vi "Get_IP_Number.vi"() -> (0 "Computer Name":string, 1 "IP Number":string)   [LabVIEW 2013]
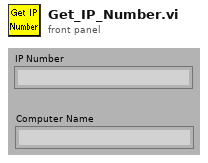
[diagram p1: front panel]
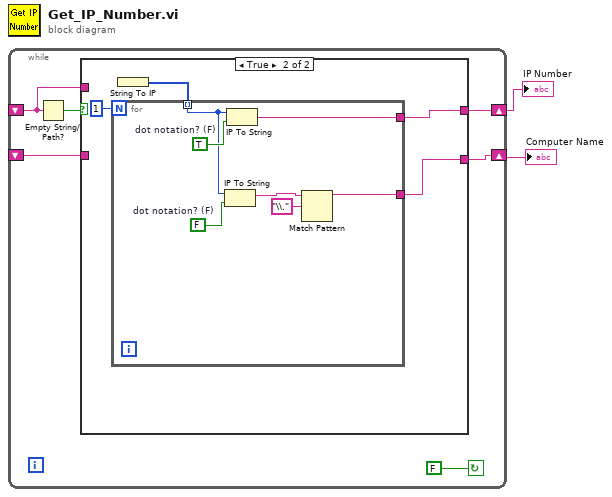
[diagram p0: block diagram]
diagram:
  n1 = while {
    shift-left: _ -> [w7]
    shift-right: [w8] -> w2
    shift-right: [w5] -> w1
    shift-left: _ -> [w4]
    stop <- FALSE continue-if-true
    n2 = Empty String/Path?(string/path=w7) -> (empty?=w3:bool)
    n3 = case shown="True" w3 {
      tunnel: [w10 w13] -> w8
      tunnel: w7 -> [w10 _]
      tunnel: [w9 w11] -> w5
      tunnel: w4 -> [w9 _]
      frame False {
      }
      frame True {
        n4 = String To IP() -> (0:w14:u32[])  [unwired: 1 out]
        n5 = for {
          N: 1 -> [_]
          tunnel: w14 -> [w18] mode=indexing
          tunnel: [w21] -> w13
          tunnel: [w15] -> w11
          w19 = FALSE  # dot notation? (F)
          w20 = TRUE  # dot notation? (F)
          n6 = IP To String(1:w19, 2:w18) -> (0:w16:string)
          n7 = IP To String(1:w20, 2:w18) -> (0:w21:string)
          n8 = Match Pattern(string=w16, regular expression="\\.") -> (before substring=w15:string)  [unwired: 1 in, 3 out]
        }
      }
    }
  }
  "IP Number" <- w2
  "Computer Name" <- w1
